vi "Add NI-XNET CAN Hardware_Create Transmit Signal.vi"(7 "SysDef Ref":T1, 8 "error in (no error)":errorcluster, 9 "TriggerType":i32, 10 "Trigger Node Path":string, 11 "Frame Based Signal":refnum<k24>) -> (0 "error out":errorcluster, 3 "Frame Based Signal out":refnum<k24>)   [LabVIEW 2019, in "Simple SysDef API.lvlib"]
uses:
  <userlib>/SimpleSysDef/Simple SysDef API.lvlib
  <userlib>/SimpleSysDef/_SubVIs/System Definition Reference.ctl
  NationalInstruments.VeriStand.SystemDefinitionAPI
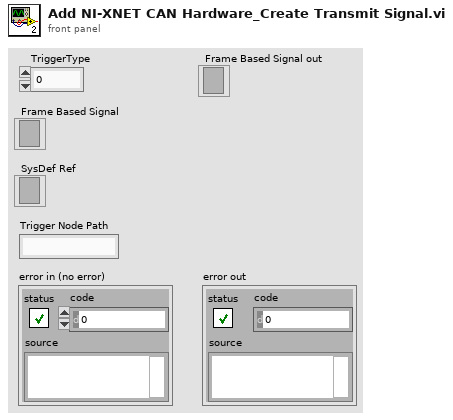
[diagram p1: front panel]
types:
  T1 = typedef "Simple SysDef API.lvlib/System Definition Reference.ctl" = refnum<k24>
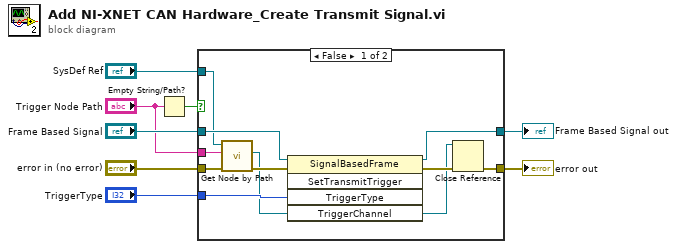
[diagram p0: block diagram]
diagram:
  n1 = Empty String/Path?(string/path="Trigger Node Path") -> (empty?=w5:bool)
  n2 = case shown="False" w5 {
    tunnel: "error in (no error)" -> [w18 w19]
    tunnel: [w17 w20] -> w1
    tunnel: [w10 w19] -> w2
    tunnel: "Frame Based Signal" -> [w15 w20]
    tunnel: "Trigger Node Path" -> [w14 _]
    tunnel: "TriggerType" -> [w13 _]
    tunnel: "SysDef Ref" -> [w12 _]
    frame False {
      n3 = call <userlib>:"Get Node by Path.vi"("error in (no error)"=w18, "System Definition Node Path"=w14, "SysDef Ref"=w12) -> ("error out"=w16:errorcluster, "Node Ref"=w9:refnum<k24>)  [unwired: 6 in, 1 out]
      n4 = invoke class="SignalBasedFrame" method="SetTransmitTrigger"(reference=w15, error in=w16, "TriggerType"=w13, "TriggerChannel"=w9) -> (reference out=w17:refnum<k24>, error out=w11:errorcluster)  [unwired: 1 in, 3 out]
      n5 = Close Reference(reference=w9, error in (no error)=w11) -> (error out=w10:errorcluster)
    }
    frame True {
    }
  }
  "error out" <- w2
  "Frame Based Signal out" <- w1
